vi "ResourceVisa.vi"() -> ()   [LabVIEW 2020]
panel:
  out "display file":string
  in  "Path":path
  out "display m3510A":string
  in  "Voltmeter Picotest M3510A":refnum<visa-resource-name>
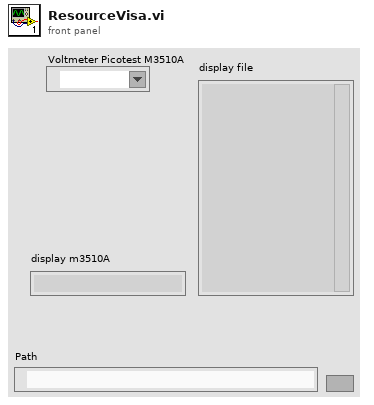
[diagram p1: front panel]
types:
  T1 = enum16{"read/write", "read-only", "write-only", ""}
  T2 = enum16{"open", "replace", "create", "open or create", "replace or create", "replace or create with confirmation", ""}
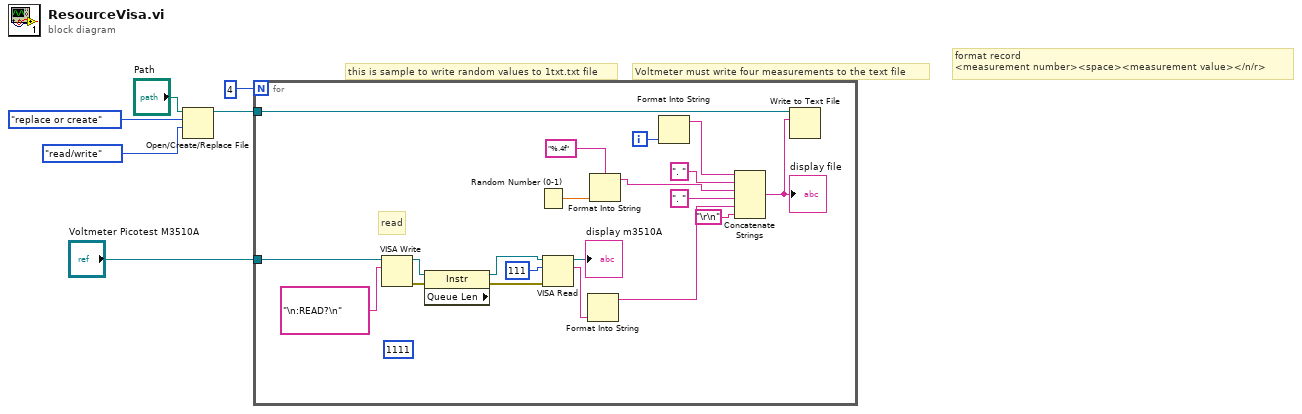
[diagram p0: block diagram]
diagram:
  # "format record \n<measurement number><space><measurement value></n/r>"
  # "Voltmeter must write four measurements to the text file"
  # "this is sample to write random values to 1txt.txt file"
  n1 = Open/Create/Replace File(file path (use dialog)="Path", operation (0:open)=T2."replace or create", access (0:read/write)=T1."read/write") -> (refnum out=w2:refnum<file>)  [unwired: 3 in, 2 out]
  n2 = for {
    N: 4 -> [_]
    tunnel: "Voltmeter Picotest M3510A" -> [w9]
    tunnel: w2 -> [w7]
    i -> [w19]
    (unwired) 1111
    # "read"
    n3 = VISA Write(VISA resource name=w9, write buffer="\n:READ?\n") -> (VISA resource name out=w24:refnum<visa-resource-name>, error out=w25:errorcluster)  [unwired: 1 in, 1 out]
    n4 = property class="Instr" props=["Queue Len"](reference=w24, error in=w25) -> (reference out=w23:refnum<visa-resource-name>, error out=w22:errorcluster)  [unwired: 1 out]
    n5 = Random Number (0-1)() -> (number: 0 to 1=w20:dbl)
    n6 = VISA Read(VISA resource name=w23, byte count=111, error in (no error)=w22) -> (VISA resource name out=→"display m3510A":refnum<visa-resource-name>, read buffer=w10:string)  [unwired: 2 out]
    n7 = Format Into String(w10) -> (resulting string=w12:string)  [unwired: 3 in, 1 out]
    n8 = Format Into String(format string="%.4f", w20) -> (resulting string=w16:string)  [unwired: 2 in, 1 out]
    n9 = Format Into String(w19) -> (resulting string=w18:string)  [unwired: 3 in, 1 out]
    n10 = Concatenate Strings(w18, ". ", w16, ". ", w12, "\r\n") -> (w8:string)
    "display file" <- w8
    n11 = Write to Text File(file (use dialog)=w7, text=w8) -> ()  [unwired: 2 in, 3 out]
  }
